vi "Cluster_Get Attributes.vi"(8 "error in (no error)":errorcluster, 11 "Cluster In":refnum<class "Cluster.lvclass">) -> (0 "error out":errorcluster, 2 "Cluster Attributes":T1, 3 "Cluster Out":refnum<class "Cluster.lvclass">)   [LabVIEW 2017, in "Front Panel Publisher.lvlib" / "Cluster.lvclass"]
uses:
  Cluster.lvclass
  Attributes.ctl
  Object_class/Object.lvclass
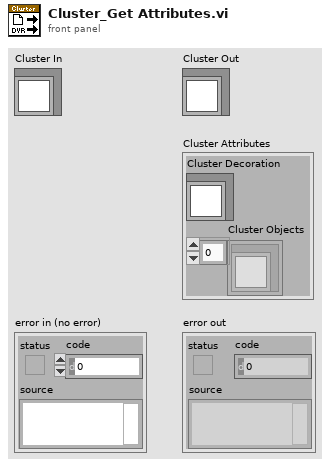
[diagram p1: front panel]
types:
  T1 = typedef "Front Panel Publisher.lvlib/Cluster.lvclass/Attributes.ctl" = cluster{"Cluster Decoration":refnum<class "Object.lvclass">, "Cluster Objects":refnum<class "Object.lvclass">[]}
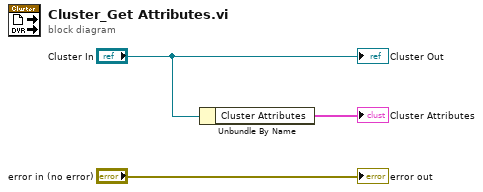
[diagram p0: block diagram]
diagram:
  n1 = Unbundle By Name("Cluster In") -> ("Cluster Attributes"=→"Cluster Attributes":T1)
  "error out" <- "error in (no error)"
  "Cluster Out" <- "Cluster In"
